vi "Engine Control Test.vi"(3 "Input buffer":T1, 4 "Sequence Context":T2) -> (0 "error out":errorcluster, 1 "Test Data":T3 {"Numeric Measurement" format="%.2f"})   [LabVIEW 2013]
uses:
  <vilib>/addons/TestStand/_TSLegacy.llb/LabVIEW Test - Test Data.ctl
  <vilib>/addons/TestStand/_TSLegacy.llb/LabVIEW Test - Sequence Context.ctl
  SupportVIs.llb/LabVIEW Test - Input Buffer.ctl
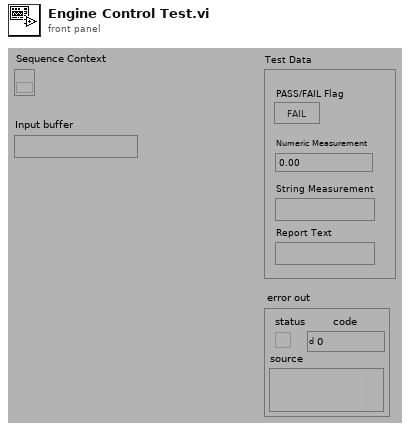
[diagram p1: front panel]
types:
  T1 = typedef "LabVIEW Test - Input Buffer.ctl" = string
  T2 = typedef "LabVIEW Test - Sequence Context.ctl" = refnum<k7>
  T3 = typedef "LabVIEW Test - Test Data.ctl" = cluster{"PASS/FAIL Flag":bool, "Numeric Measurement":dbl, "String Measurement":string, "Report Text":string}
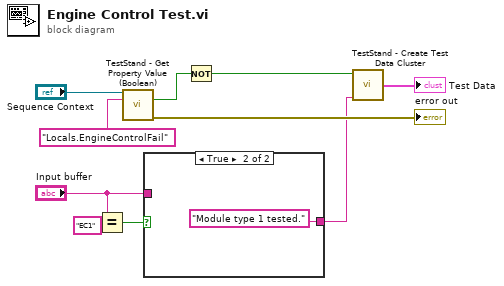
[diagram p0: block diagram]
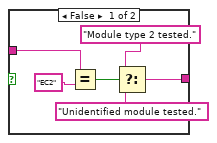
[diagram p2: hidden frame]
diagram:
  n1 = Equal?(x="Input buffer", y="EC1") -> (x = y?=w3:bool)
  n2 = call "TestStand - Get Property Value (Boolean).vi"("Sequence Context In"="Sequence Context", "Lookup String"="Locals.EngineControlFail") -> ("Value"=w7:bool, "error out"=→"error out":errorcluster)  [unwired: 1 in, 11 out]
  n3 = case shown="True" w3 {
    tunnel: "Input buffer" -> [w16 _]
    tunnel: [w11 "Module type 1 tested." ("y")] -> w1
    frame False {
      n4 = Equal?(x=w16, y="EC2") -> (x = y?=w14:bool)
      n5 = Select(t="Module type 2 tested." ("y"), s=w14, f="Unidentified module tested." ("y")) -> (s? t:f=w11:string)
    }
    frame True {
    }
  }
  n6 = Not(x=w7) -> (.not. x?=w5:bool)
  n7 = call "TestStand - Create Test Data Cluster.vi"("Report Text"=w1, "PASS/FAIL Flag"=w5) -> ("Test Data"=→"Test Data":T3)  [unwired: 2 in]
